vi "Register for Laser Events.vi"(8 "error in (no error)":errorcluster, 11 "Laser Controller in":refnum<class "Laser Controller.lvclass">) -> (0 "error out":errorcluster, 1 "Laser Process State":refnum<event-registration>, 2 "Laser State":refnum<event-registration>, 3 "Laser Controller out":refnum<class "Laser Controller.lvclass">)   [LabVIEW 2022 SP3, in "Laser Controller.lvclass"]
uses:
  Laser Controller.lvclass
  Laser State Data/Events.ctl
  Laser State Data/Laser State.ctl
  Laser State Data/Time and Temp.ctl
  XY Stage/Process Actor/Process Framework/Process State Data/Events.ctl
  Laser Controller.lvclass/Laser Controller.ctl
  Laser State Data/Laser State Data.lvclass/Laser State Data.ctl
  Laser State Data/Read Events.vi
  XY Stage/Process Actor/Process Framework/Process State Data/Process State Data.lvclass
  Laser State Data/Laser State Data.lvclass
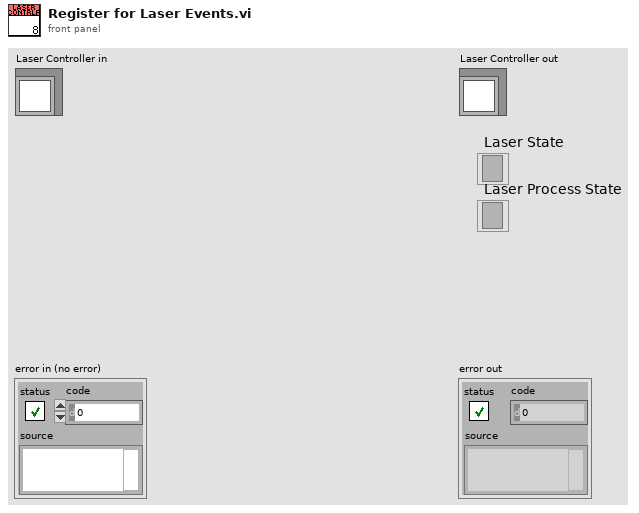
[diagram p1: front panel]
types:
  T1 = typedef "Laser State Data.lvclass/Events.ctl" = cluster{"Temp":refnum<user-event>, "Current Power":refnum<user-event>, "Laser State":refnum<user-event>, "Time and Temp":refnum<user-event>}
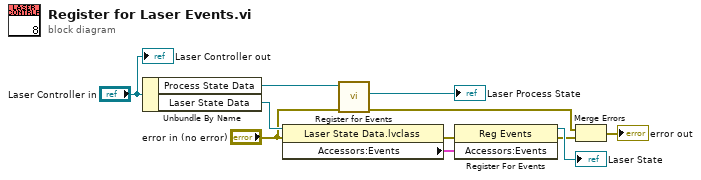
[diagram p0: block diagram]
diagram:
  n1 = Unbundle By Name("Laser Controller in") -> ("Process State Data"=w10:refnum<data-value>, "Laser State Data"=w9:refnum<data-value>)
  n2 = property class="Laser State Data.lvclass"(reference=w9, error in="error in (no error)") -> (error out=w4:errorcluster, "Accessors:Events"=w8:T1)  [unwired: 1 out]
  n3 = call "Register for Events.vi"("error in (no error)"="error in (no error)", "Process State"=w10) -> ("error out"=w3:errorcluster, "Event Registration Refnum"=→"Laser Process State":refnum<event-registration>)  [unwired: 7 in, 1 out]
  n4 = register-events(error in=w4, w8) -> (reference out=→"Laser State":refnum<event-registration>, error out=w2:errorcluster)  [unwired: 1 in]
  n5 = Merge Errors(w3, w2) -> (→"error out":errorcluster)
  "Laser Controller out" <- "Laser Controller in"
